vi "Process Image.vi"(8 "error in (no error)":errorcluster, 9 "Saturation (counts)":dbl=256.0 format="%#_13g", 10 "Image Analysis IN":T1, 11 "Cluster in":T3={"Crosshair IN"={"Draw"=TRUE, "Target"={"x"=20.0, "y"=20.0}, "Size"={"x"=20.0, "y"=20.0}, "Angle"=1250067.0, "Color"=1250067, "Thickness"=20, "CrosshairLabel"=""}, "Autoscale"=FALSE, "Scale"={"scale factor"=0.0, "Scale"=FALSE}, "Lowpass IN"={"LowPass"=FALSE, "Size & Tolerance"={"X Size"=0, "Y Size"=0, "% Tolerance"=0}}, "Image"=refnum, "GUI_centroid overlay"={"CentroidX array"=[], "CentroidY array"=[], "CentroidX"=0.0, "CentroidY"=0.0, "# images to average"=1250067, "Crosshair"={"Draw"=TRUE, "Target"={"x"=20.0, "y"=20.0}, "Size"={"x"=20.0, "y"=20.0}, "Angle"=1250067.0, "Color"=1250067, "Thickness"=20, "CrosshairLabel"=""}}, "GUI Crosshair"={"Draw"=TRUE, "Target"={"x"=20.0, "y"=20.0}, "Size"={"x"=20.0, "y"=20.0}, "Angle"=1250067.0, "Color"=1250067, "Thickness"=20, "CrosshairLabel"=""}, "Crosshair2 IN"={"Draw"=TRUE, "Target"={"x"=20.0, "y"=20.0}, "Size"={"x"=20.0, "y"=20.0}, "Angle"=1250067.0, "Color"=1250067, "Thickness"=20, "CrosshairLabel"=""}, "calibration image"=refnum, "Perspective correection"=FALSE, "Background image"=refnum, "Subtract background"=FALSE, "Rotate Image"={"Rotate"=FALSE, "Rotation Angle"=0.0}} {"Crosshair2 IN"."Thickness" max=0; "Crosshair2 IN"."Target"."y" min=0.0 max=0.0; "Crosshair2 IN"."Target"."x" min=0.0 max=0.0; "Crosshair2 IN"."Angle" format="%#_13g"; "Crosshair2 IN"."Size"."y" min=0.0 max=0.0; "Crosshair2 IN"."Size"."x" min=0.0 max=0.0; "GUI Crosshair"."Thickness" max=0; "GUI Crosshair"."Target"."y" min=0.0 max=0.0; "GUI Crosshair"."Target"."x" min=0.0 max=0.0; "GUI Crosshair"."Angle" format="%#_13g"; "GUI Crosshair"."Size"."y" min=0.0 max=0.0; "GUI Crosshair"."Size"."x" min=0.0 max=0.0; "GUI_centroid overlay"."Crosshair"."Thickness" max=0; "GUI_centroid overlay"."Crosshair"."Target"."y" min=0.0 max=0.0; "GUI_centroid overlay"."Crosshair"."Target"."x" min=0.0 max=0.0; "GUI_centroid overlay"."Crosshair"."Angle" format="%#_13g"; "GUI_centroid overlay"."Crosshair"."Size"."y" min=0.0 max=0.0; "GUI_centroid overlay"."Crosshair"."Size"."x" min=0.0 max=0.0; "Crosshair IN"."Thickness" max=0; "Crosshair IN"."Target"."y" min=0.0 max=0.0; "Crosshair IN"."Target"."x" min=0.0 max=0.0; "Crosshair IN"."Angle" format="%#_13g"; "Crosshair IN"."Size"."y" min=0.0 max=0.0; "Crosshair IN"."Size"."x" min=0.0 max=0.0}) -> (0 "error out":errorcluster, 1 "Perspective correction error":bool, 2 "Image Analysis OUT":T1, 3 "Cluster out":T3={"Crosshair IN"={"Draw"=TRUE, "Target"={"x"=20.0, "y"=20.0}, "Size"={"x"=20.0, "y"=20.0}, "Angle"=1250067.0, "Color"=1250067, "Thickness"=20, "CrosshairLabel"=""}, "Autoscale"=FALSE, "Scale"={"scale factor"=0.0, "Scale"=FALSE}, "Lowpass IN"={"LowPass"=FALSE, "Size & Tolerance"={"X Size"=0, "Y Size"=0, "% Tolerance"=0}}, "Image"=refnum, "GUI_centroid overlay"={"CentroidX array"=[], "CentroidY array"=[], "CentroidX"=0.0, "CentroidY"=0.0, "# images to average"=1250067, "Crosshair"={"Draw"=TRUE, "Target"={"x"=20.0, "y"=20.0}, "Size"={"x"=20.0, "y"=20.0}, "Angle"=1250067.0, "Color"=1250067, "Thickness"=20, "CrosshairLabel"=""}}, "GUI Crosshair"={"Draw"=TRUE, "Target"={"x"=20.0, "y"=20.0}, "Size"={"x"=20.0, "y"=20.0}, "Angle"=1250067.0, "Color"=1250067, "Thickness"=20, "CrosshairLabel"=""}, "Crosshair2 IN"={"Draw"=TRUE, "Target"={"x"=20.0, "y"=20.0}, "Size"={"x"=20.0, "y"=20.0}, "Angle"=1250067.0, "Color"=1250067, "Thickness"=20, "CrosshairLabel"=""}, "calibration image"=refnum, "Perspective correection"=FALSE, "Background image"=refnum, "Subtract background"=FALSE, "Rotate Image"={"Rotate"=FALSE, "Rotation Angle"=0.0}} {"Crosshair2 IN"."Thickness" max=0; "Crosshair2 IN"."Target"."y" min=0.0 max=0.0; "Crosshair2 IN"."Target"."x" min=0.0 max=0.0; "Crosshair2 IN"."Angle" format="%#_13g"; "Crosshair2 IN"."Size"."y" min=0.0 max=0.0; "Crosshair2 IN"."Size"."x" min=0.0 max=0.0; "GUI Crosshair"."Thickness" max=0; "GUI Crosshair"."Target"."y" min=0.0 max=0.0; "GUI Crosshair"."Target"."x" min=0.0 max=0.0; "GUI Crosshair"."Angle" format="%#_13g"; "GUI Crosshair"."Size"."y" min=0.0 max=0.0; "GUI Crosshair"."Size"."x" min=0.0 max=0.0; "GUI_centroid overlay"."Crosshair"."Thickness" max=0; "GUI_centroid overlay"."Crosshair"."Target"."y" min=0.0 max=0.0; "GUI_centroid overlay"."Crosshair"."Target"."x" min=0.0 max=0.0; "GUI_centroid overlay"."Crosshair"."Angle" format="%#_13g"; "GUI_centroid overlay"."Crosshair"."Size"."y" min=0.0 max=0.0; "GUI_centroid overlay"."Crosshair"."Size"."x" min=0.0 max=0.0; "Crosshair IN"."Thickness" max=0; "Crosshair IN"."Target"."y" min=0.0 max=0.0; "Crosshair IN"."Target"."x" min=0.0 max=0.0; "Crosshair IN"."Angle" format="%#_13g"; "Crosshair IN"."Size"."y" min=0.0 max=0.0; "Crosshair IN"."Size"."x" min=0.0 max=0.0})   [LabVIEW 2020]
uses:
  Controls/Image Processing Controls.ctl
  Controls/Crosshair type def.ctl
  <vilib>/vision/Image Controls.llb/IMAQ Image.ctl
  Controls/GUI_running average centroid overlay.ctl
  Controls/Image Analysis Controls.ctl
  <vilib>/vision/NI_Vision_Development_Module.lvlib
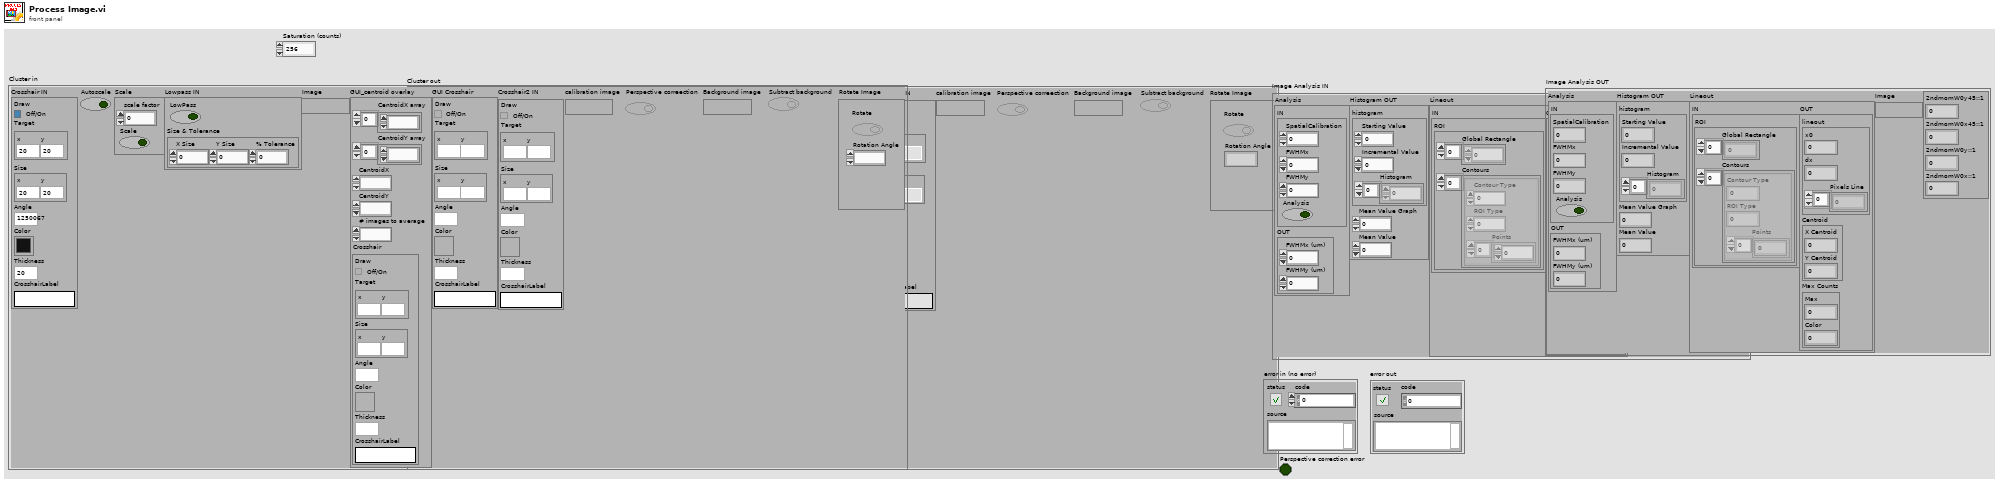
[diagram p1: front panel]
types:
  T1 = typedef "Image Analysis Controls.ctl" = cluster{"Analysis":cluster{"IN":cluster{"SpatialCalibration":dbl, "FWHMx":dbl, "FWHMy":dbl, "Analysis":bool}, "OUT":cluster{"FWHMx (um)":dbl, "FWHMy (um)":dbl}}, "Histogram OUT":cluster{"histogram":cluster{"Starting Value":sgl, "Incremental Value":sgl, "Histogram":u32[]}, "Mean Value Graph":sgl, "Mean Value":sgl}, "Lineout":cluster{"IN":cluster{"ROI":cluster{"Global Rectangle":i32[], "Contours":cluster{"Contour Type":u32, "ROI Type":u32, "Points":i32[]}[]}}, "OUT":cluster{"lineout":cluster{"x0":sgl, "dx":sgl, "Pixels Line":sgl[]}, "Centroid":cluster{"X Centroid":sgl, "Y Centroid":sgl}, "Max Counts":cluster{"Max":sgl, "Color":u32}}}, "Image":T2, "variables":cluster{"2ndmomW0y45::1":dbl, "2ndmomW0x45::1":dbl, "2ndmomW0y::1":dbl, "2ndmomW0x::1":dbl}}
  T2 = typedef "IMAQ Image.ctl" = refnum<image>
  T3 = typedef "Image Processing Controls.ctl" = cluster{"Crosshair IN":T4, "Autoscale":bool, "Scale":cluster{"scale factor":dbl, "Scale":bool}, "Lowpass IN":cluster{"LowPass":bool, "Size & Tolerance":cluster{"X Size":i32, "Y Size":i32, "% Tolerance":i32}}, "Image":T2, "GUI_centroid overlay":T5, "GUI Crosshair":T4, "Crosshair2 IN":T4, "calibration image":T2, "Perspective correection":bool, "Background image":T2, "Subtract background":bool, "Rotate Image":cluster{"Rotate":bool, "Rotation Angle":dbl}}
  T4 = typedef "Crosshair type def.ctl" = cluster{"Draw":bool, "Target":cluster{"x":dbl, "y":dbl}, "Size":cluster{"x":dbl, "y":dbl}, "Angle":dbl, "Color":u32, "Thickness":u8, "CrosshairLabel":string}
  T5 = typedef "GUI_running average centroid overlay.ctl" = cluster{"CentroidX array":dbl[], "CentroidY array":dbl[], "CentroidX":dbl, "CentroidY":dbl, "# images to average":i32, "Crosshair":T4}
  T6 = cluster{"LowPass":bool, "Size & Tolerance":cluster{"X Size":i32, "Y Size":i32, "% Tolerance":i32}}
  T7 = cluster{"SpatialCalibration":dbl, "FWHMx":dbl, "FWHMy":dbl, "Analysis":bool}
  T8 = cluster{"ROI":cluster{"Global Rectangle":i32[], "Contours":cluster{"Contour Type":u32, "ROI Type":u32, "Points":i32[]}[]}}
  T9 = cluster{"histogram":cluster{"Starting Value":sgl, "Incremental Value":sgl, "Histogram":u32[]}, "Mean Value Graph":sgl, "Mean Value":sgl}
  T10 = cluster{"lineout":cluster{"x0":sgl, "dx":sgl, "Pixels Line":sgl[]}, "Centroid":cluster{"X Centroid":sgl, "Y Centroid":sgl}, "Max Counts":cluster{"Max Value":sgl, "Color":u32}}
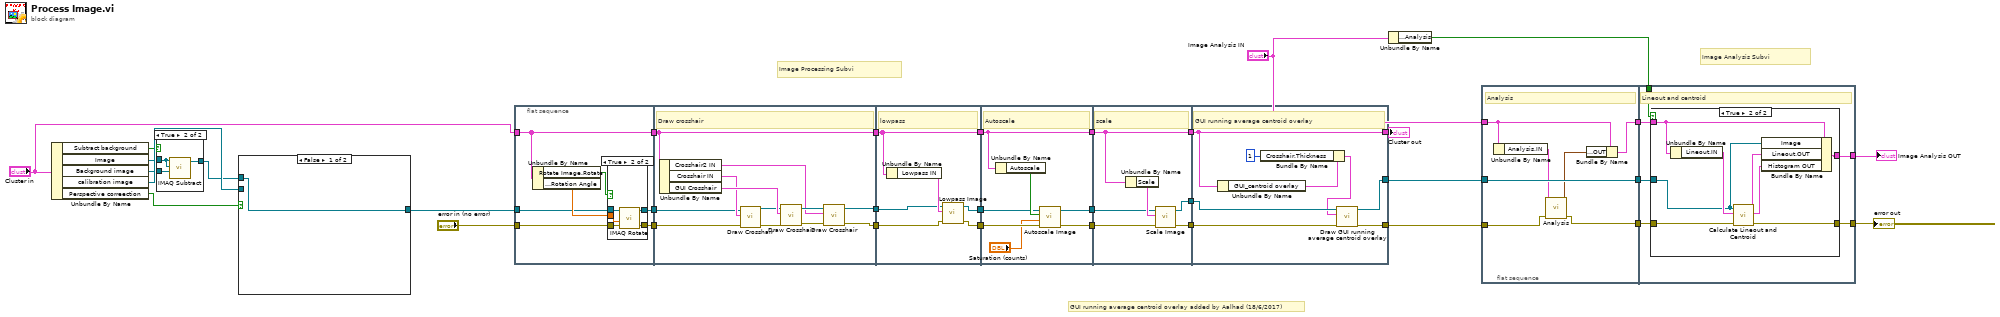
[diagram p0: block diagram]
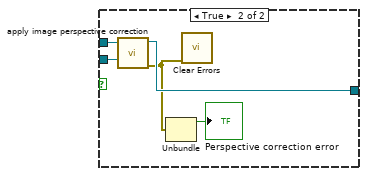
[diagram p3: hidden frame]
diagram:
  # "GUI running average centroid overlay added by Aalhad (18/6/2017)"
  # "Image Analysis Subvi"
  # "Image Processing Subvi"
  n1 = Unbundle By Name("Cluster in") -> ("Subtract background"=w5:bool, "Image"=w6:T2, "Background image"=w4:T2, "calibration image"=w10:T2, "Perspective correection"=w8:bool)
  n2 = case shown="True" w5 {
    tunnel: [w35 w38] -> w7
    tunnel: w6 -> [w35 w37]
    tunnel: w4 -> [_ w36]
    frame False {
    }
    frame True {
      n3 = call "IMAQ Subtract"("Image Src A"=w37, "Image Dst"=w37, "Image Src B"=w36) -> ("Image Dst Out"=w38:T2)  [unwired: 4 in, 1 out]
    }
  }
  n4 = case shown="False" w8 {
    tunnel: w7 -> [w39 w44]
    tunnel: w10 -> [_ w43]
    tunnel: [w39 w42] -> w9
    frame False {
    }
    frame True {
      n5 = call "apply image perspective correction.vi"("Calibration Image"=w43, "Image To Correct"=w44) -> ("error out"=w41:errorcluster, "Corrected Image"=w42:T2)  [unwired: 8 in]
      n6 = Unbundle(w41) -> ("status"=→"Perspective correction error":bool)  [unwired: 2 out]
      n7 = call <vilib>:"Clear Errors.vi"("error in (no error)"=w41) -> ()  [unwired: 5 in, 2 out]
    }
  }
  n8 = flat-sequence {
    tunnel: w9 -> [w48]
    tunnel: "error in (no error)" -> [w46]
    tunnel: "Cluster in" -> [w51]
    tunnel: [w51] -> w3
    tunnel: [w47] -> w2
    tunnel: [w45] -> w1
    tunnel: [w70] -> w29
    tunnel: [w64] -> w28
    tunnel: [w62] -> w22
    tunnel: w3 -> [w70]
    tunnel: w2 -> [w59]
    tunnel: w1 -> [w69]
    tunnel: [w75] -> w34
    tunnel: [w72] -> w33
    tunnel: w29 -> [w75]
    tunnel: w28 -> [w71]
    tunnel: w22 -> [w74]
    tunnel: [w73] -> w21
    tunnel: w34 -> [w78]
    tunnel: [w78] -> w32
    tunnel: w33 -> [w82]
    tunnel: [w81] -> w31
    tunnel: w21 -> [w79]
    tunnel: [w80] -> w20
    tunnel: w32 -> [w85]
    tunnel: w31 -> [w88]
    tunnel: w20 -> [w84]
    tunnel: [w85] -> w18
    tunnel: [w87] -> w17
    tunnel: [w86] -> w16
    tunnel: [w97] -> w26
    tunnel: [w96] -> w25
    tunnel: [w94] -> w30
    tunnel: w18 -> [w94]
    tunnel: w17 -> [w95]
    tunnel: w16 -> [w93]
    frame #0 {
      n9 = Unbundle By Name(w51) -> ("Rotate Image.Rotate"=w49:bool, "Rotate Image.Rotation Angle"=w50:dbl)
      n10 = case shown="True" w49 {
        tunnel: w50 -> [_ w58]
        tunnel: w48 -> [w53 w57]
        tunnel: [w53 w56] -> w47
        tunnel: w46 -> [w52 w55]
        tunnel: [w52 w54] -> w45
        frame False {
        }
        frame True {
          n11 = call "IMAQ Rotate"("error in (no error)"=w55, "Angle (degrees)"=w58, "Image Src"=w57) -> ("error out"=w54:errorcluster, "Image Dst Out"=w56:T2)  [unwired: 7 in]
        }
      }
    }
    frame #1 {
      # "Draw crosshair"
      n12 = Unbundle By Name(w70) -> ("Crosshair2 IN"=w60:T4, "Crosshair IN"=w61:T4, "GUI Crosshair"=w68:T4)
      n13 = call "Draw Crosshair.vi"("error in"=w69, "Crosshair"=w61, "Image in"=w59) -> ("error out"=w66:errorcluster, "image out"=w67:T2)  [unwired: 7 in]
      n14 = call "Draw Crosshair.vi"("error in"=w66, "Crosshair"=w68, "Image in"=w67) -> ("error out"=w65:errorcluster, "image out"=w63:T2)  [unwired: 7 in]
      n15 = call "Draw Crosshair.vi"("error in"=w65, "Crosshair"=w60, "Image in"=w63) -> ("error out"=w64:errorcluster, "image out"=w62:T2)  [unwired: 7 in]
    }
    frame #2 {
      # "lowpass"
      n16 = Unbundle By Name(w75) -> ("Lowpass IN"=w76:T6)
      n17 = call "Lowpass Image.vi"("error in"=w71, "Lowpass IN"=w76, "Refnum in"=w74) -> ("error out"=w72:errorcluster, "Refnum out"=w73:T2)  [unwired: 7 in]
    }
    frame #3 {
      # "Autoscale"
      n18 = Unbundle By Name(w78) -> ("Autoscale"=w83:bool)
      n19 = call "Autoscale Image.vi"("error in (no error)"=w82, "Saturation (counts)"="Saturation (counts)", "Autoscale"=w83, "Refnum in"=w79) -> ("error out"=w81:errorcluster, "Refnum out"=w80:T2)  [unwired: 6 in]
    }
    frame #4 {
      # "scale"
      n20 = Unbundle By Name(w85) -> ("Scale"=w89:cluster{"scale factor":dbl, "Scale":bool})
      n21 = call "Scale Image.vi"("error in (no error)"=w88, "Scale"=w89, "Refnum in"=w84) -> ("error out"=w87:errorcluster, "Refnum out"=w86:T2)  [unwired: 7 in]
    }
    frame #5 {
      # "GUI running average centroid overlay"
      n22 = Unbundle By Name(w94) -> ("GUI_centroid overlay"=w91:T5)
      n23 = Bundle By Name(cluster=w91, "Crosshair.Thickness"=u8 1) -> (w90:T5)
      n24 = call "Draw GUI running average centroid overlay.vi"("error in"=w95, "GUI_centroid overlay"=w90, "Image in"=w93) -> ("error out"=w96:errorcluster, "image out"=w97:T2)  [unwired: 7 in]
    }
  }
  n25 = Unbundle By Name("Image Analysis IN") -> ("Analysis.IN.Analysis"=w12:bool)
  n26 = flat-sequence {
    tunnel: w25 -> [w102]
    tunnel: w26 -> [w104]
    tunnel: "Image Analysis IN" -> [w100]
    tunnel: [w99] -> w15
    tunnel: [w104] -> w14
    tunnel: [w101] -> w13
    tunnel: w15 -> [w108]
    tunnel: w14 -> [w110]
    tunnel: w13 -> [w109]
    tunnel: [w107] -> w23
    tunnel: [w106] -> w24
    tunnel: w12 -> [w105]
    frame #0 {
      # "Analysis"
      n27 = Unbundle By Name(w100) -> ("Analysis.IN"=w103:T7)
      n28 = call "Analysis.vi"("error in"=w102, "IN"=w103) -> ("error out"=w101:errorcluster, "OUT"=w98:cluster{"FWHMx (um)":dbl, "FWHMy (um)":dbl})  [unwired: 8 in]
      n29 = Bundle By Name(cluster=w100, "Analysis.OUT"=w98) -> (w99:T1)
    }
    frame #1 {
      # "Lineout and centroid"
      n30 = case shown="True" w105 {
        tunnel: w110 -> [_ w118]
        tunnel: w109 -> [w112 w117]
        tunnel: w108 -> [w111 w116]
        tunnel: [w111 w114] -> w107
        tunnel: [w112 w113] -> w106
        frame False {
        }
        frame True {
          n31 = Unbundle By Name(w116) -> ("Lineout.IN"=w120:T8)
          n32 = call "Calculate Lineout and Centroid.vi"("error in (no error)"=w117, "Lineout IN"=w120, "Image"=w118) -> ("error out"=w113:errorcluster, "Histogram OUT"=w115:T9, "Lineout Out"=w119:T10)  [unwired: 6 in]
          n33 = Bundle By Name(cluster=w116, "Image"=w118, "Lineout.OUT"=w119, "Histogram OUT"=w115) -> (w114:T1)
        }
      }
    }
  }
  "Cluster out" <- w30
  "error out" <- w24
  "Image Analysis OUT" <- w23
